vi "PPMS.Get Helium Level.vi"(8 "error in (no error)":errorcluster, 11 "instrument.PPMS":refnum<class "instrument.PPMS.lvclass">) -> (0 "error out":errorcluster, 2 "Helium Level (%)":dbl, 3 "instrument.PPMS out":refnum<class "instrument.PPMS.lvclass">)   [LabVIEW 2019, in "instrument.PPMS.lvclass"]
uses:
  instrument.PPMS.lvclass
  instrument.PPMS.lvclass/instrument.PPMS.ctl
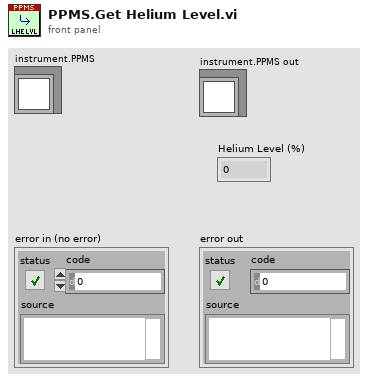
[diagram p1: front panel]
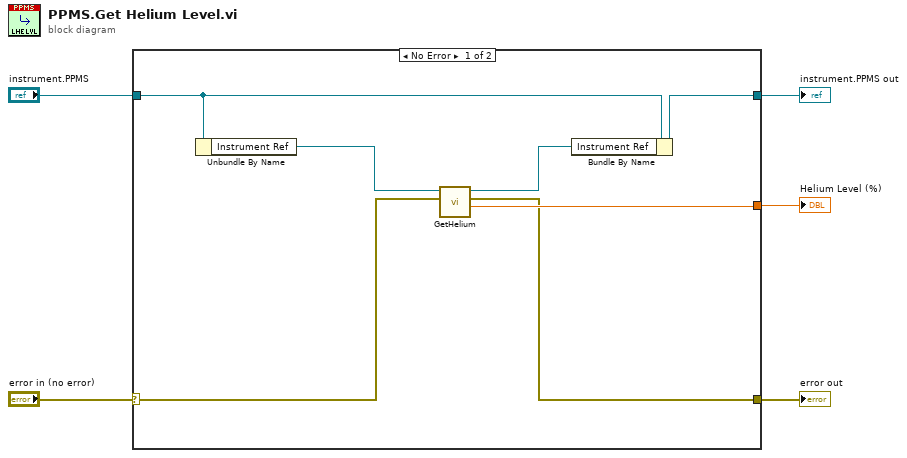
[diagram p0: block diagram]
diagram:
  n1 = case shown="No Error" "error in (no error)" {
    selector: "error in (no error)" -> [w6 w14]
    tunnel: [w10 w14] -> w5
    tunnel: "instrument.PPMS" -> [w7 w13]
    tunnel: [w8 w13] -> w2
    tunnel: [w11 _] -> w1
    frame No Error {
      n2 = Unbundle By Name(w7) -> ("Instrument Ref"=w12:refnum<k24>)
      n3 = call "GetHelium.vi"("error in (no error)"=w6, "Instrument Refnum in"=w12) -> ("Helium Level (%)"=w11:dbl, "error out"=w10:errorcluster, "Instrument Ref Out"=w9:refnum<k24>)  [unwired: 3 in]
      n4 = Bundle By Name(cluster=w7, "Instrument Ref"=w9) -> (w8:refnum<class "instrument.PPMS.lvclass">)
    }
    frame Error {
    }
  }
  "Helium Level (%)" <- w1
  "error out" <- w5
  "instrument.PPMS out" <- w2
